vi "Enqueue Data.vi"(8 "error in (no error)":errorcluster, 10 "Message Data":T1) -> (0 "error out":errorcluster)   [LabVIEW 2023, in "Controller.lvlib"]
doc: "VI used to enqueue data to be used in the module."
uses:
  Controller.lvlib
  Type Def/FGV Queue State.ctl
  Type Def/Message Data.ctl
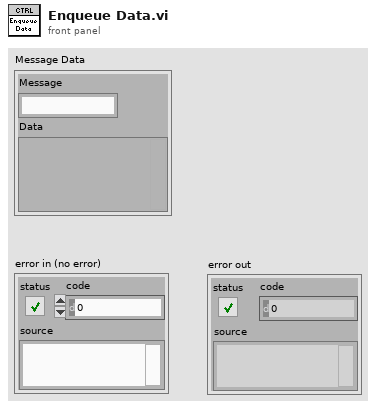
[diagram p1: front panel]
types:
  T1 = typedef "Controller.lvlib/Message Data.ctl" = cluster{"Message":string, "Data":variant}
  T2 = typedef "Controller.lvlib/FGV Queue State.ctl" = enum16{"Get", "Set"}
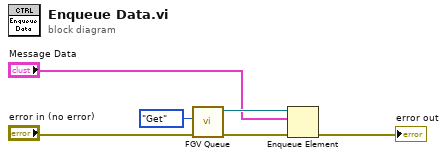
[diagram p0: block diagram]
diagram:
  n1 = call "FGV Queue.vi"("error in (no error)"="error in (no error)", "FGV Queue State"=FGV_Queue_State."Get") -> ("error out"=w3:errorcluster, "queue out"=w4:refnum<queue>)  [unwired: 8 in]
  n2 = Enqueue Element(queue=w4, element="Message Data", error in (no error)=w3) -> (error out=→"error out":errorcluster)  [unwired: 1 in, 2 out]
